vi "CompressAndUpdate(IMAQ Image).vi"(7 "force CVT update (false)":bool, 8 "error in":errorcluster, 10 "IMAQ Image":T1, 11 "command or variable name":string) -> (0 "error out":errorcluster)   [LabVIEW 2011]
uses:
  IMAQ Image.ctl
panel:
  out "time for compression":u32(graph)
  in  "precision (6)":i16
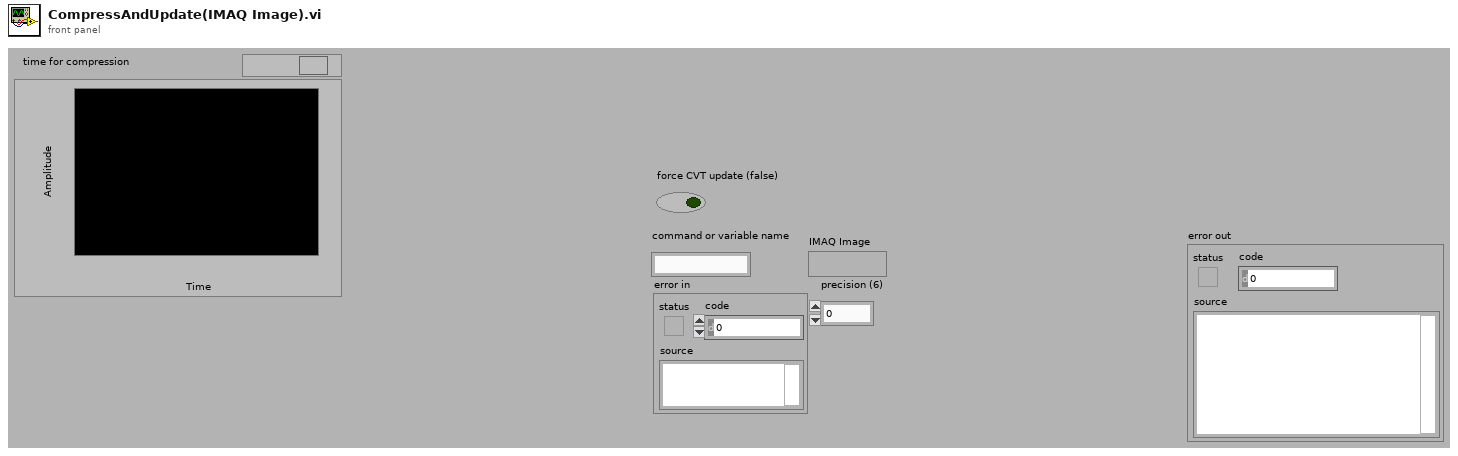
[diagram p1: front panel]
types:
  T1 = typedef "IMAQ Image.ctl" = refnum<image>
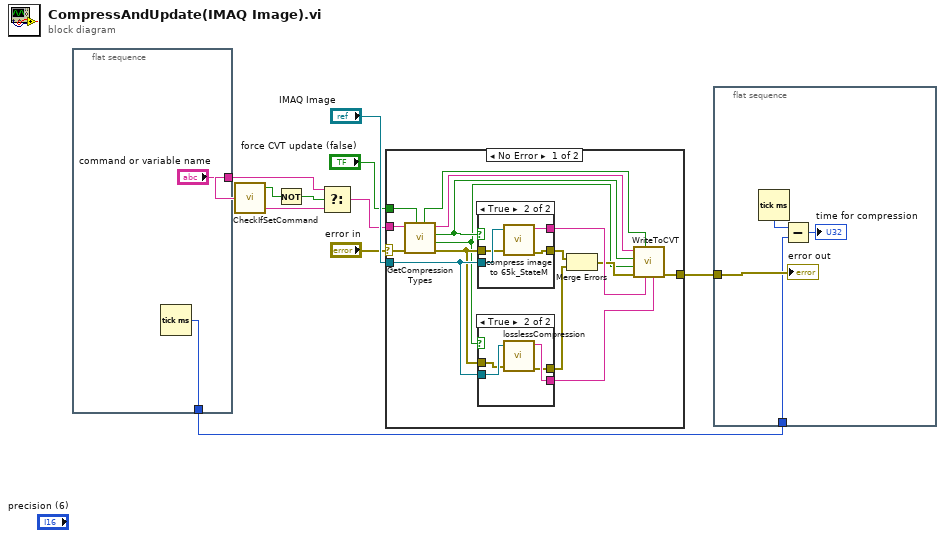
[diagram p0: block diagram]
diagram:
  n1 = flat-sequence {
    tunnel: ["command or variable name"] -> w4
    tunnel: [w11] -> w1
    frame #0 {
      n2 = Tick Count (ms)() -> (millisecond timer value=w11:u32)
    }
  }
  n3 = call "CheckIfSetCommand.vi"("Command"=w4) -> ("setCommand?"=w5:bool, "variable"=w7:string)  [unwired: 1 out]
  n4 = Not(x=w5) -> (.not. x?=w6:bool)
  n5 = Select(t=w4, s=w6, f=w7) -> (s? t:f=w3:string)
  n6 = case shown="No Error" "error in" {
    selector: "error in" -> [w26 w38]
    tunnel: [w15 w38] -> w10
    tunnel: w3 -> [w27 _]
    tunnel: "IMAQ Image" -> [w24 _]
    tunnel: "force CVT update (false)" -> [w25 _]
    frame No Error {
      n7 = call "GetCompressionTypes.vi"("force CVT update"=w25, "error in"=w26, "variable"=w27) -> ("error out"=w23:errorcluster, "non compressed"=w13:bool, "compressed"=w14:bool, "variable out"=w16:string, "force CVT update out"=w17:bool)  [unwired: 4 in]
      n8 = case shown="True" w14 {
        tunnel: w24 -> [_ w35]
        tunnel: [_ w37] -> w20
        tunnel: w23 -> [w33 w34]
        tunnel: [w33 w36] -> w22
        frame False {
        }
        frame True {
          n9 = call "compress image to 65k_StateM.vi"("Image"=w35, "error in (no error)"=w34) -> ("Data String"=w37:string, "error out"=w36:errorcluster)  [unwired: 4 in]
        }
      }
      n10 = case shown="True" w13 {
        tunnel: w24 -> [_ w32]
        tunnel: [_ w31] -> w19
        tunnel: w23 -> [w28 w30]
        tunnel: [w28 w29] -> w21
        frame False {
        }
        frame True {
          n11 = call "losslessCompression.vi"("Image"=w32, "error in (no error)"=w30) -> ("Data String"=w31:string, "error out"=w29:errorcluster)  [unwired: 4 in]
        }
      }
      n12 = Merge Errors(w22, w21) -> (w18:errorcluster)
      n13 = call "WriteToCVT.vi"("non compressed string"=w19, "compressed string"=w20, "force CVT update"=w17, "error in"=w18, "non compressed"=w13, "compressed"=w14, "variable"=w16) -> ("error out"=w15:errorcluster)  [unwired: 4 in]
    }
    frame Error {
    }
  }
  n14 = flat-sequence {
    tunnel: w10 -> [w42]
    tunnel: w1 -> [w39]
    frame #0 {
      n15 = Tick Count (ms)() -> (millisecond timer value=w41:u32)
      n16 = Subtract(x=w41, y=w39) -> (x-y=→"time for compression":u32)
      "error out" <- w42
    }
  }
